vi "SLM.vi"(8 "Stopp":bool, 10 "SLOT":i32=100 min=0 max=999 step=100, 11 "USB":i32) -> ()   [LabVIEW 2020]
doc: "This VI provides a GUI for SLM modules. It implements an abstract module interface, where callers provide the only necessary and sufficient information for callee modules via the datafields USB, SLOT and Stopp. All module intern information are handled hidden by the module. Thereby, a caller must not \"know\" about such internals."
panel:
  in  "ZeroBtn":bool caption="Boolean"
  in  "Pulsed Mode":bool
  in  "Intensity":sgl min=0 max=100 step=1 format="%.1f"
  out "Head Type":string
  in  "Trigger Source":u16(ring) items=["80 MHz (int.)", "40 MHz (int.)", "20 MHz (int.)", "10 MHz (int.)", " 5 MHz (int.)", " 2.5 MHz (int.)", "rising  edge (ext.)", "falling edge (ext.)"]
  # "%"
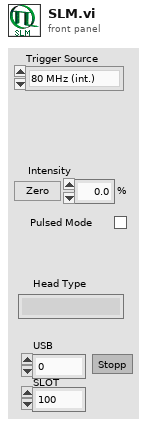
[diagram p1: front panel]
types:
  T1 = cluster{"Freq":i32, "PulseMode":u8, "HeadType":i32}
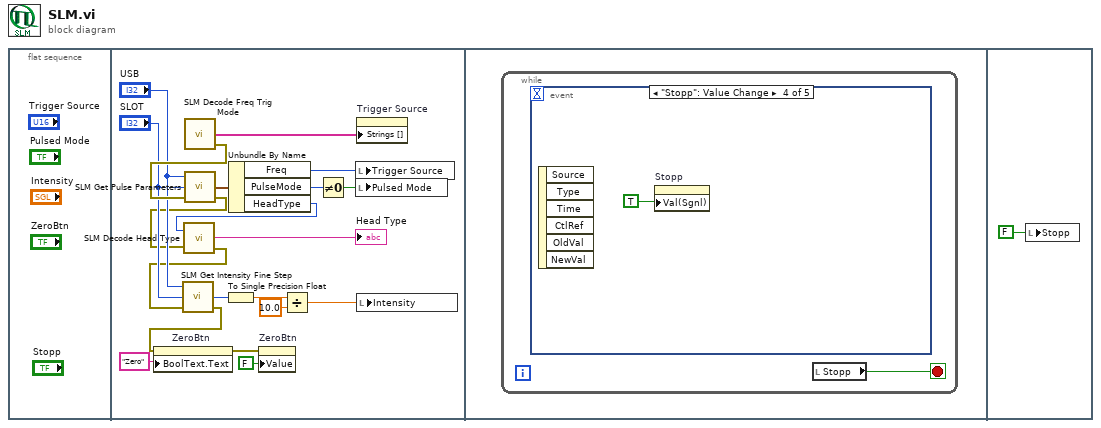
[diagram p0: block diagram]
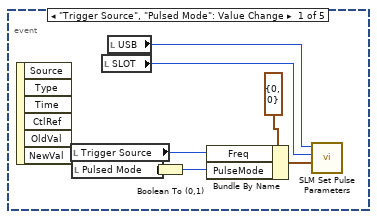
[diagram p2: hidden frame]
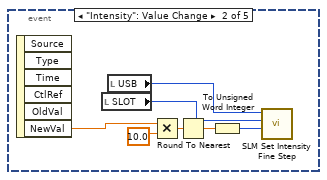
[diagram p3: hidden frame]
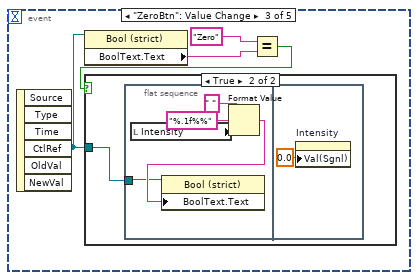
[diagram p4: hidden frame]
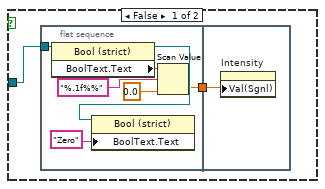
[diagram p5: hidden frame]
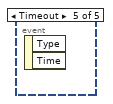
[diagram p6: hidden frame]
diagram:
  n1 = flat-sequence {
    frame #0 {
    }
    frame #1 {
      n2 = call "SLM Decode Freq Trig Mode.vi"() -> ("FreqTrigMode"=w20:string[], "error out"=w16:errorcluster)  [unwired: 2 in, 1 out]
      n3 = call "SLM Get Pulse Parameters.vi"("error in (no error)"=w16, "SlotId"="SLOT", "DevIdx"="USB") -> ("error out"=w10:errorcluster, "SLM Pulse Parameters"=w17:T1)  [unwired: 1 out]
      n4 = Unbundle By Name(w17) -> ("Freq"=w14:i32, "PulseMode"=w13:u8, "HeadType"=w12:i32)
      n5 = call "SLM Decode Head Type.vi"("HeadType"=w12, "error in (no error)"=w10) -> ("HeadType"=→"Head Type":string, "error out"=w9:errorcluster)  [unwired: 1 out]
      n6 = call "SLM Get Intensity Fine Step.vi"("error in (no error)"=w9, "SlotId"="SLOT", "DevIdx"="USB") -> ("error out"=w3:errorcluster, "Intensity"=w4:u16)  [unwired: 1 out]
      n7 = property on="ZeroBtn" class="Bool (strict)"(error in=w3, "BoolText.Text"="Zero" ("Boolean Text.Text")) -> (error out=w2:errorcluster)  [unwired: 1 in, 1 out]
      n8 = To Single Precision Float(number=w4) -> (single precision float=w7:sgl)
      n9 = property on="ZeroBtn" class="Bool (strict)"(error in=w2, "Value"=FALSE) -> ()  [unwired: 1 in, 2 out]
      n10 = Divide(x=w7, y=sgl 10.0) -> (x/y=w6:sgl)
      n11 = Not Equal To 0?(x=w13) -> (x != 0?=w18:bool)
      n12 = local write "Trigger Source"(w14) -> ()
      n13 = local write "Pulsed Mode"(w18) -> ()
      n14 = property on="Trigger Source" class="Ring (strict)"("Strings []"=w20) -> ()  [unwired: 2 in, 2 out]
      n15 = local write "Intensity"(w6) -> ()
    }
    frame #2 {
      n16 = while {
        stop <- w21 stop-if-true
        n17 = event shown="[3] \"Stopp\": Value Change" {
          selector: _ -> [_ _ _ _ _]
          dyn-events: _ -> [_ _ _ _ _]
          timeout: _ -> [_ _ _ _ _]
          event "Trigger Source", "Pulsed Mode": Value Change {
            n18 = event-data() -> ()  [unwired: 1 in, 6 out]
            n19 = local read "Trigger Source"() -> (w27:u16)
            n20 = local read "Pulsed Mode"() -> (w26:bool)
            n21 = local read "SLOT"() -> (w23:i32)
            n22 = local read "USB"() -> (w24:i32)
            n23 = Boolean To (0,1)(Boolean=w26) -> (0, 1=w25:i16)
            n24 = Bundle By Name(cluster=cluster{"Freq":i32, "PulseMode":u8} {"Freq"=0, "PulseMode"=0} ("SLM Parameter"), "Freq"=w27, "PulseMode"=w25) -> (w22:cluster{"Freq":i32, "PulseMode":u8})
            n25 = call "SLM Set Pulse Parameters.vi"("SLM Pulse Parameters"=w22, "SlotId"=w23, "DevIdx"=w24) -> ()  [unwired: 1 in, 2 out]
          }
          event "Intensity": Value Change {
            n26 = event-data() -> ("NewVal"=w29:sgl)  [unwired: 1 in, 5 out]
            n27 = local read "SLOT"() -> (w34:i32)
            n28 = local read "USB"() -> (w33:i32)
            n29 = Multiply(x=w29, y=sgl 10.0) -> (x*y=w35:sgl)
            n30 = Round To Nearest(number=w35) -> (nearest integer value=w31:sgl)
            n31 = To Unsigned Word Integer(number=w31) -> (unsigned 16bit integer=w32:u16)
            n32 = call "SLM Set Intensity Fine Step.vi"("Intensity"=w32, "SlotId"=w34, "DevIdx"=w33) -> ()  [unwired: 1 in, 2 out]
          }
          event "ZeroBtn": Value Change {
            n33 = event-data() -> ("CtlRef"=w36:refnum<vi>)  [unwired: 1 in, 5 out]
            n34 = property class="Bool (strict)"(reference=w36) -> ("BoolText.Text"=w38:string)  [unwired: 1 in, 2 out]
            n35 = Equal?(x="Zero" ("Boolean Text.Text"), y=w38) -> (x = y?=w37:bool)
            n36 = case shown="True" w37 {
              tunnel: w36 -> [w41 w50]
              frame False {
                n37 = flat-sequence {
                  tunnel: w41 -> [w48]
                  tunnel: [w43] -> w40
                  tunnel: w40 -> [w49]
                  frame #0 {
                    n38 = property class="Bool (strict)"(reference=w48) -> (reference out=w45:refnum<vi>, "BoolText.Text"=w47:string)  [unwired: 1 in, 1 out]
                    n39 = property class="Bool (strict)"(reference=w45, "BoolText.Text"="Zero" ("Boolean Text.Text")) -> ()  [unwired: 1 in, 2 out]
                    n40 = Scan Value(string=w47, format string="%.1f%%", default (0 dbl)=0.0) -> (value=w43:dbl)  [unwired: 1 out]
                  }
                  frame #1 {
                    n41 = property on="Intensity" class="DigNum (strict)"("Val(Sgnl)"=w49) -> ()  [unwired: 2 in, 2 out]
                  }
                }
              }
              frame True {
                n42 = flat-sequence {
                  tunnel: w50 -> [w51]
                  frame #0 {
                    n43 = local read "Intensity"() -> (w53:sgl)
                    n44 = Format Value(string ("")=" ", format string="%.1f%%", value (0)=w53) -> (output string=w52:string)
                    n45 = property class="Bool (strict)"(reference=w51, "BoolText.Text"=w52) -> ()  [unwired: 1 in, 2 out]
                  }
                  frame #1 {
                    n46 = property on="Intensity" class="DigNum (strict)"("Val(Sgnl)"=sgl 0.0 ("Intensity")) -> ()  [unwired: 2 in, 2 out]
                  }
                }
              }
            }
          }
          event "Stopp": Value Change {
            n47 = event-data() -> ()  [unwired: 1 in, 6 out]
            n48 = property on="Stopp" class="Bool (strict)"("Val(Sgnl)"=TRUE ("Value (Signaling)")) -> ()  [unwired: 2 in, 2 out]
          }
          event Timeout {
            n49 = event-data() -> ()  [unwired: 1 in, 2 out]
          }
        }
        n50 = local read "Stopp"() -> (w21:bool)
      }
    }
    frame #3 {
      n51 = local write "Stopp"(FALSE ("Stopp")) -> ()
    }
  }
